vi "fromDevULong64.vi"(1 "argin":u64) -> (0 "ArgIO":cluster{"num data":u8[], "str data":string[]})   [LabVIEW 2014, in "tango.lvlib"]
uses:
  tango.lvlib
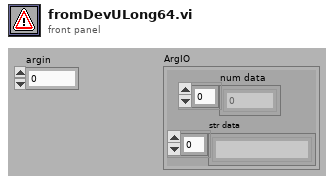
[diagram p1: front panel]
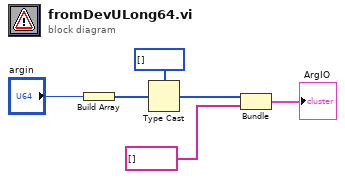
[diagram p0: block diagram]
diagram:
  n1 = Build Array("argin") -> (w1:u64[])
  n2 = Type Cast(type=u8[] [], x=w1) -> (*(type *) &x=w3:u8[])
  n3 = Bundle(w3, string[] []) -> (→"ArgIO":cluster{u8[], string[]})  [unwired: 1 in]
